vi "test display matrix to array.vi"() -> ()   [LabVIEW 2018]
panel:
  out "spreadsheet string":string
  in  "Display in":string[][](array[string])=array41x201[8241 elements]
  out "Display array 2":string[][](array[string])
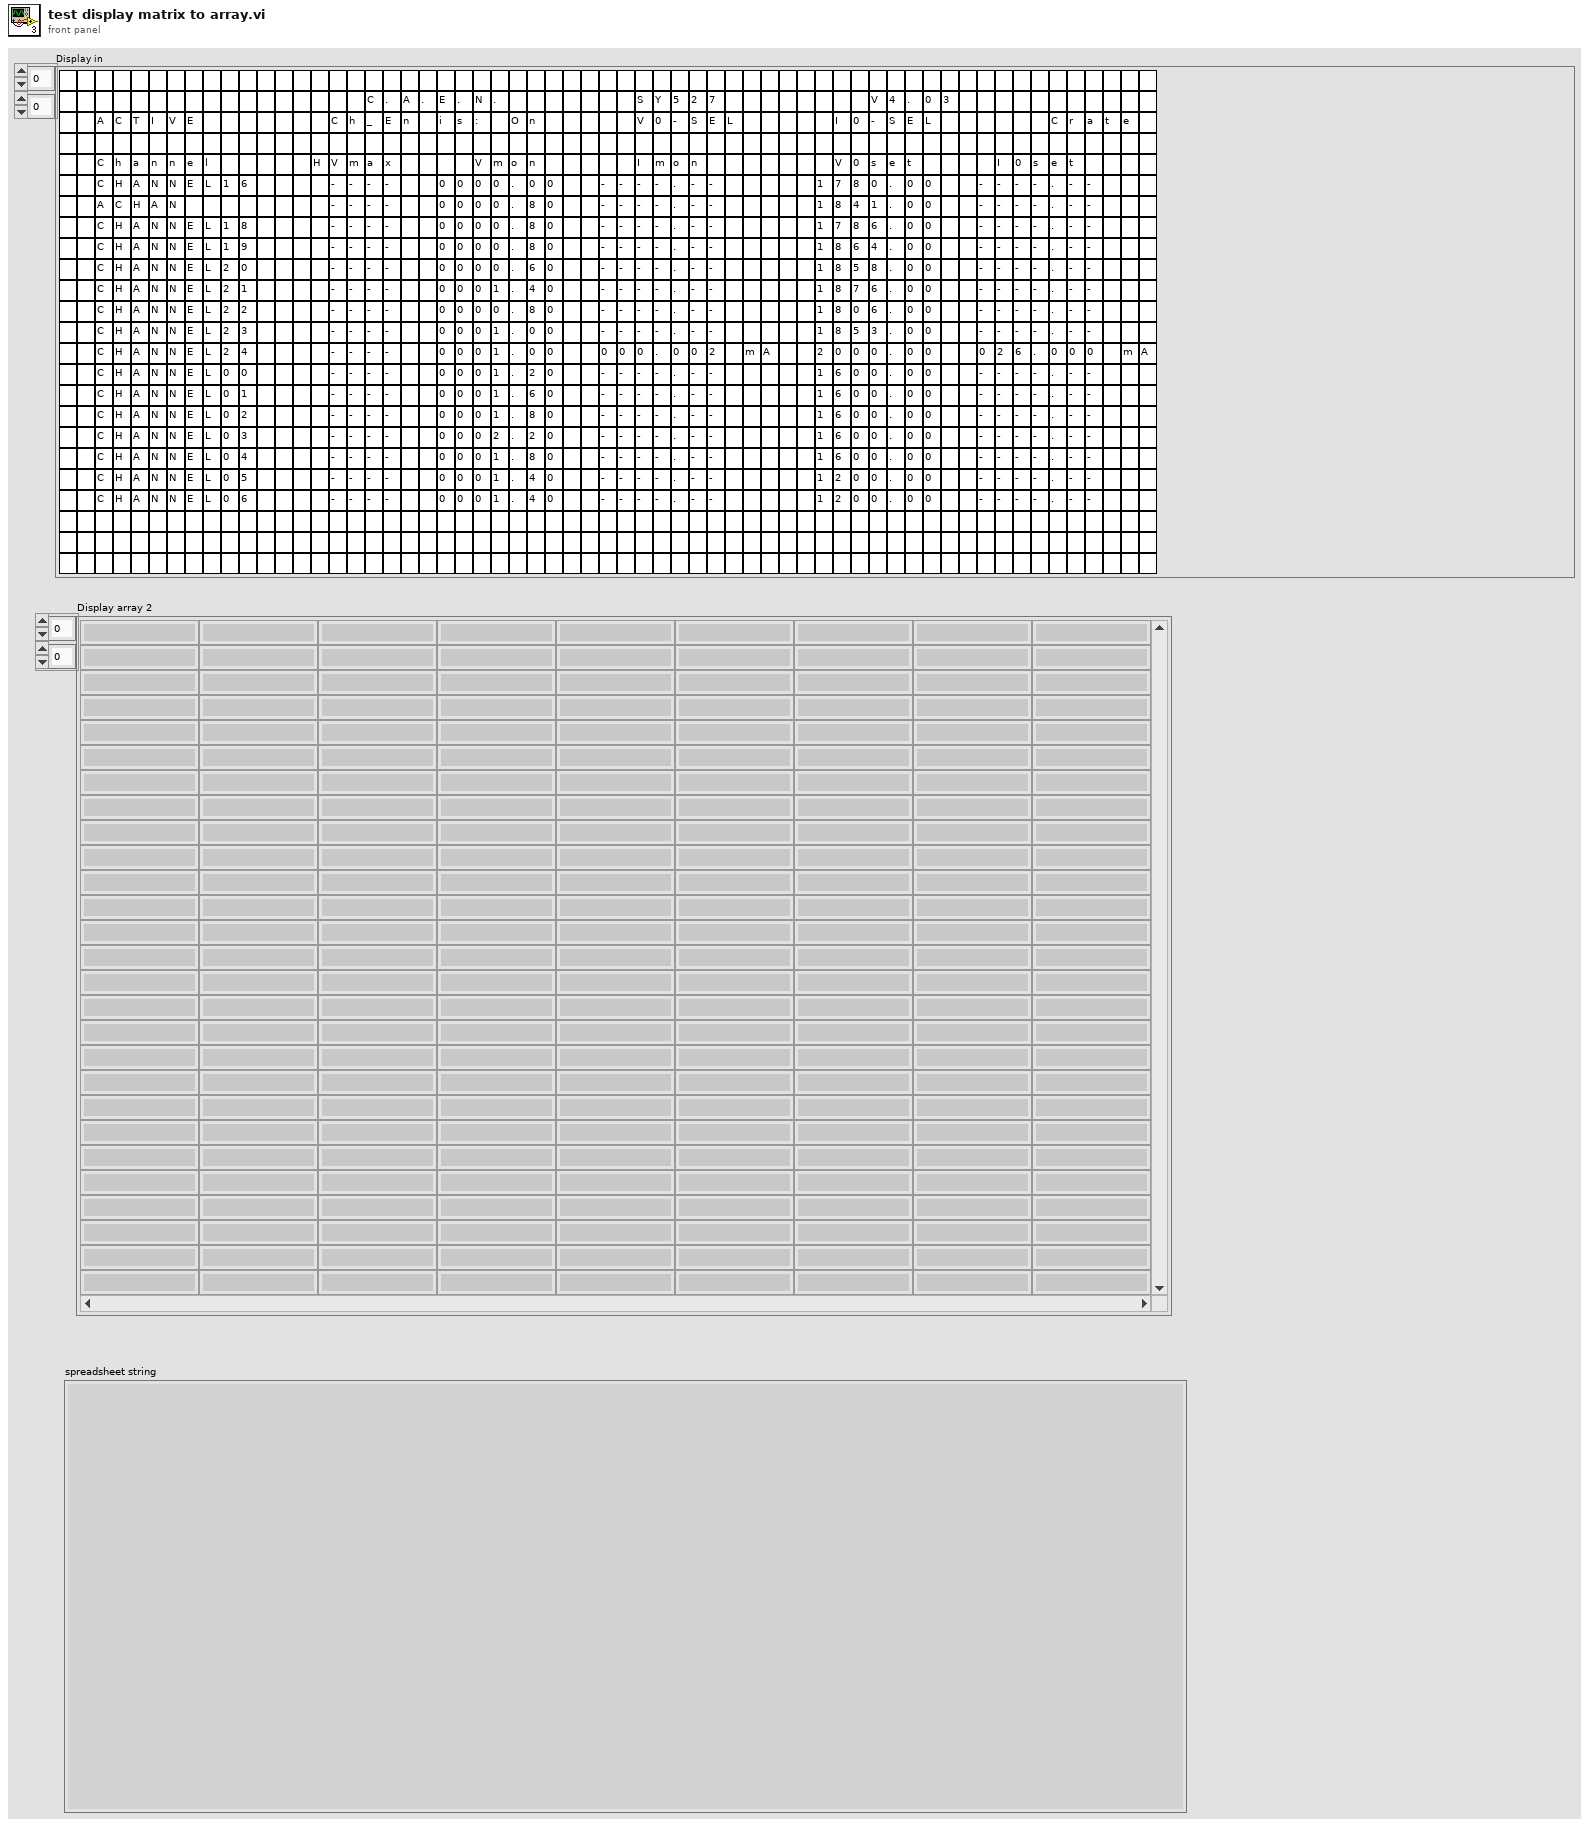
[diagram p1: front panel]
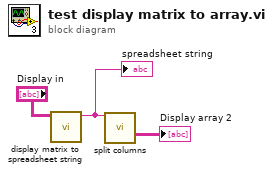
[diagram p0: block diagram]
diagram:
  n1 = call "display matrix to spreadsheet string.vi"("Display"="Display in") -> ("spreadsheet string"=w2:string)  [unwired: 7 in, 3 out]
  "spreadsheet string" <- w2
  n2 = call "split columns.vi"("Display string"=w2) -> ("Array"=→"Display array 2":string[][])  [unwired: 10 in, 4 out]
